vi "Do.vi"(8 "error in (no error)":errorcluster, 10 "Actor In":refnum<class "Actor.lvclass">, 11 "Nested Status Message in":refnum<class "Nested Status Message.lvclass">) -> (0 "error out":errorcluster, 1 "Stop Actor":bool, 2 "Actor Out":refnum<class "Actor.lvclass">)   [LabVIEW 2020, in "Artifex.lvlib" / "Nested Status Message.lvclass"]
uses:
  Nested Status Message.lvclass
  Actor/Actor.lvclass
  Actor Status Handler/Actor Status Handler.lvclass
  Nested Status Message.lvclass/Nested Status Message.ctl
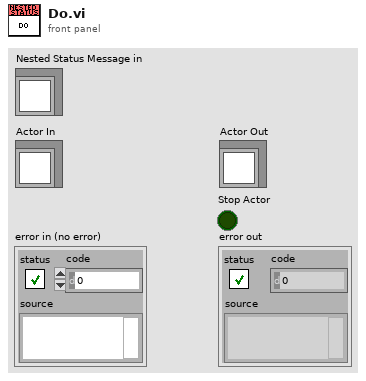
[diagram p1: front panel]
types:
  T1 = typedef "Artifex.lvlib/Actor State.ctl" = enum16{"Error", "Initialized", "Started", "Closing", "Closed"}
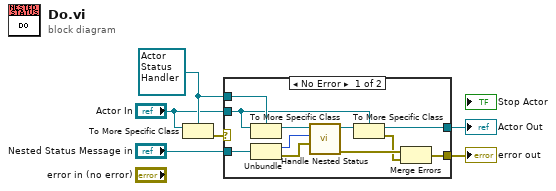
[diagram p0: block diagram]
diagram:
  w5 = refnum<class "Actor Status Handler.lvclass"> refnum ("Artifex.lvlib:Actor Status Handler.lvclass")
  n1 = To More Specific Class(target class=w5, reference="Actor In") -> (error out=w6:errorcluster)  [unwired: 1 in, 1 out]
  n2 = case shown="No Error" w6 {
    selector: w6 -> [_ w18]
    tunnel: "Actor In" -> [w10 w19]
    tunnel: w5 -> [w17 _]
    tunnel: "Nested Status Message in" -> [w15 _]
    tunnel: [w11 w19] -> w2
    tunnel: [w7 w18] -> w1
    frame No Error {
      n3 = To More Specific Class(target class=w17, reference=w10) -> (specific class reference=w16:refnum<class "Actor Status Handler.lvclass">)  [unwired: 1 in, 1 out]
      n4 = Unbundle(w15) -> (w14:T1, w13:errorcluster)
      n5 = call-dynamic "Handle Nested Status.vi"("Actor Error"=w13, "State"=w14, "Actor Status Handler in"=w16) -> ("error out"=w9:errorcluster, "Actor Status Handler out"=w12:refnum<class "Actor Status Handler.lvclass">)  [unwired: 7 in]
      n6 = To More Specific Class(target class=w10, reference=w12) -> (specific class reference=w11:refnum<class "Actor.lvclass">, error out=w8:errorcluster)  [unwired: 1 in]
      n7 = Merge Errors(w9, w8) -> (w7:errorcluster)
    }
    frame Error {
    }
  }
  "error out" <- w1
  "Actor Out" <- w2
